vi "solar Msg Voyager (Relay).vi"(8 "error in (no error)":errorcluster, 9 "CMD_DATA":variant, 10 "CMD":string, 11 "solar in":refnum<class "solar.lvclass">) -> (0 "error out":errorcluster, 3 "solar out":refnum<class "solar.lvclass">)   [LabVIEW 2018]
doc: "This relays any local SOLAR message back to COSMOS by checking if the 'HDR_GUID' attribute is included in the CMD_DATA. If the 'HDR_GUID' attribute is not found, this assumes the command is a local command and the command is relayed."
uses:
  solar.lvclass
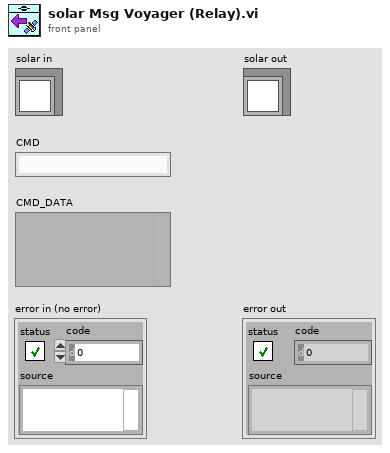
[diagram p1: front panel]
types:
  T1 = typedef "solar_voy_ctl Voyager Refnum.ctl" = refnum<k1>
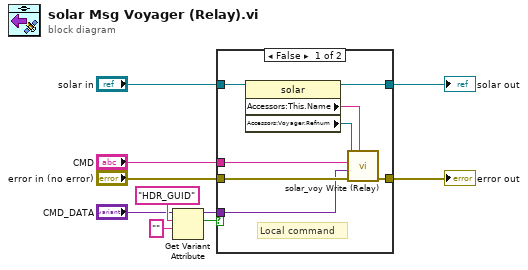
[diagram p0: block diagram]
diagram:
  n1 = Get Variant Attribute(Variant="CMD_DATA", name="HDR_GUID", default value (empty Variant)="") -> (duplicate Variant=w2:variant, found=w1:bool)  [unwired: 1 in, 2 out]
  n2 = case shown="False" w1 {
    tunnel: [w18 w20] -> w10
    tunnel: [w15 w19] -> w9
    tunnel: "error in (no error)" -> [w14 w19]
    tunnel: "CMD" -> [w13 _]
    tunnel: "solar in" -> [w12 w20]
    tunnel: w2 -> [w11 _]
    frame False {
      # "Local command"
      n3 = property class="solar"(reference=w12) -> (reference out=w18:refnum<class "solar.lvclass">, "Accessors:This.Name"=w16:string, "Accessors:Voyager.Refnum"=w17:T1)  [unwired: 1 in, 1 out]
      n4 = call "solar_voy Write (Relay).vi"("TARGET"=w16, "error in (no error)"=w14, "Variant (No HDR)"=w11, "PACKET"=w13, "Voyager Refnum in"=w17) -> ("error out"=w15:errorcluster)  [unwired: 5 in, 1 out]
    }
    frame True {
      # "Remote command\n- Do not relay"
    }
  }
  "error out" <- w9
  "solar out" <- w10
